vi "Day 6.1.vi"(11 "input":string[](array[string])) -> (3 "ouptut part 1":u64)   [LabVIEW 2021]
uses:
  <vilib>/regexp/Match Regular Expression.xnode
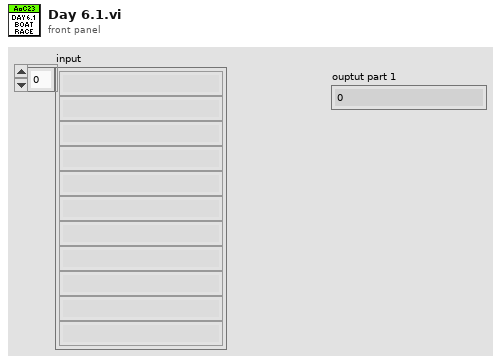
[diagram p1: front panel]
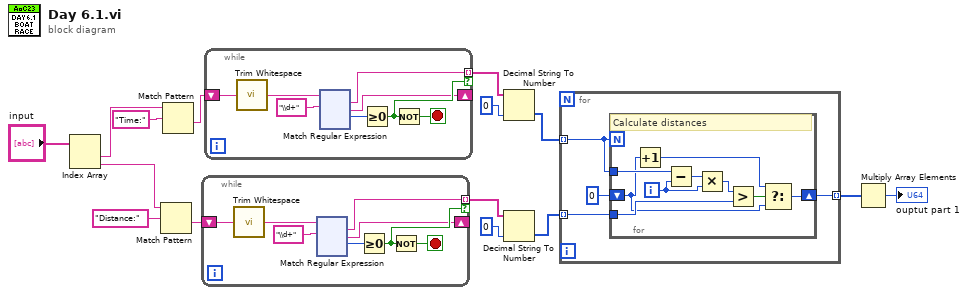
[diagram p0: block diagram]
diagram:
  n1 = Index Array(array="input") -> (element #1=w14:string, element #2=w11:string)  [unwired: 2 in]
  n2 = Match Pattern(string=w11, regular expression="Distance:") -> (after substring=w9:string)  [unwired: 1 in, 3 out]
  n3 = Match Pattern(string=w14, regular expression="Time:") -> (after substring=w10:string)  [unwired: 1 in, 3 out]
  n4 = while {
    tunnel: [w17] -> w6 mode=indexing if=w20
    shift-right: [w18] -> _
    shift-left: w9 -> [w23]
    stop <- w19 stop-if-true
    n5 = call <vilib>:"Trim Whitespace.vi"("string"=w23) -> ("trimmed string"=w16:string)  [unwired: 1 in]
    n6 = xnode "Match Regular Expression"("input string"=w16, "regular expression"="\\d+") -> ("whole match"=w17:string, "after match"=w18:string, "offset past match"=w21:i32)  [unwired: 4 in, 2 out]
    n7 = Greater Or Equal To 0?(x=w21) -> (x >= 0?=w20:bool)
    n8 = Not(x=w20) -> (.not. x?=w19:bool)
  }
  n9 = while {
    tunnel: [w142] -> w8 mode=indexing if=w145
    shift-right: [w143] -> _
    shift-left: w10 -> [w148]
    stop <- w144 stop-if-true
    n10 = call <vilib>:"Trim Whitespace.vi"("string"=w148) -> ("trimmed string"=w141:string)  [unwired: 1 in]
    n11 = xnode "Match Regular Expression"("input string"=w141, "regular expression"="\\d+") -> ("whole match"=w142:string, "after match"=w143:string, "offset past match"=w146:i32)  [unwired: 4 in, 2 out]
    n12 = Greater Or Equal To 0?(x=w146) -> (x >= 0?=w145:bool)
    n13 = Not(x=w145) -> (.not. x?=w144:bool)
  }
  n14 = Decimal String To Number(string=w8, default (0L)=u64 0 ("default (0 I32)")) -> (number=w4:u64[])  [unwired: 1 in, 1 out]
  n15 = Decimal String To Number(string=w6, default (0L)=u64 0 ("default (0 I32)")) -> (number=w3:u64[])  [unwired: 1 in, 1 out]
  n16 = for {
    tunnel: w4 -> [w269] mode=indexing
    tunnel: w3 -> [w268] mode=indexing
    tunnel: [w266] -> w2 mode=indexing
    n17 = for {
      N: w269 -> [_]
      tunnel: w269 -> [w278]
      tunnel: w268 -> [w274]
      shift-right: [w272] -> w266
      shift-left: u64 0 -> [w270]
      i -> [w276]
      # "Calculate distances"
      n18 = Increment(x=w270) -> (x+1=w271:u64)
      n19 = Subtract(x=w278, y=w276) -> (x-y=w277:u64)
      n20 = Multiply(x=w277, y=w276) -> (x*y=w275:u64)
      n21 = Greater?(x=w275, y=w274) -> (0:w273:bool)
      n22 = Select(t=w271, s=w273, f=w270) -> (s? t:f=w272:u64)
    }
  }
  n23 = Multiply Array Elements(1:w2) -> (0:→"ouptut part 1":u64)
